vi "nanocal -- nuclear schottky fit -- 2x2 -- V9.vi"() -> ()   [LabVIEW 2021] (continued)
              n225 = for {
                tunnel: w525 -> [w532] mode=indexing
                tunnel: w524 -> [w533]
                tunnel: w523 -> [w531]
                tunnel: [w529] -> w522 mode=indexing
                n226 = Look In Map(map=w533, key=w532) -> (value=w530:string)  [unwired: 1 in, 1 out]
                n227 = Concatenate Strings(w531, w530) -> (w529:string)
              }
            }
            n228 = call "string parse mathematica list assosiated array -- V2.vi"("action"=3-lorentzian-heat-response_action."create emty string" ("derivative"), "array of IDs"=w519) -> ("string out"=w520:string)  [unwired: 8 in, 1 out]
            n229 = local write "string OUT"(w520) -> ()
          }
          frame "action: update enums" {
            w537 = map{string, string} {}  # Size: 0
            w543 = map{i32, string} {}  # Size: 0
            # "gives a key"
            n230 = local read "selector"() -> (w535:T10)
            n231 = local read "all short filenames"() -> (w538:map{string, string})
            n232 = in-place {
              w560 = map{i32, dbl} {}  # Size: 0
              w566 = map{i32, dbl} {}  # Size: 0
              w567 = map{i32, dbl} {}  # Size: 0
              w569 = map{i32, dbl} {}  # Size: 0
              w568 = map{i32, dbl} {}  # Size: 0
              n233 = in-place-cluster #4(w535) -> ("lookup.all set of"=w554:set{dbl}, "lookup.all sides"=w553:set{dbl}, "lookup.all T's"=w552:set{dbl}, "lookup.all θ's"=w551:set{dbl}, "lookup.all B's"=w550:set{dbl})  [unwired: 5 out]
              n234 = for {
                shift-right: [w573] -> w559
                shift-left: w560 -> [w574]
                tunnel: [w571] -> w561 mode=indexing
                tunnel: w554 -> [w570] mode=indexing
                i -> [w572]
                n235 = Number To Decimal String(number=w570) -> (decimal integer string=w571:string)  [unwired: 1 in]
                n236 = Insert Into Map(map in=w574, key=w572, value=w570) -> (map out=w573:map{i32, dbl})  [unwired: 2 out]
              }
              n237 = for {
                shift-right: [w584] -> w556
                shift-left: w567 -> [w585]
                tunnel: [w582] -> w563 mode=indexing
                tunnel: w552 -> [w581] mode=indexing
                i -> [w583]
                n238 = Number To Fractional String(number=w581, precision (6)=i16 3) -> (F-format string=w582:string)  [unwired: 2 in]
                n239 = Insert Into Map(map in=w585, key=w583, value=w581) -> (map out=w584:map{i32, dbl})  [unwired: 2 out]
              }
              n240 = property on="set (1T|2B)" class="Ring (strict)"("Strings []"=w561) -> ()  [unwired: 2 in, 2 out]
              n241 = property on="T (K)" class="Ring (strict)"("Strings []"=w563) -> ()  [unwired: 2 in, 2 out]
              n242 = for {
                shift-right: [w578] -> w558
                shift-left: w566 -> [w579]
                tunnel: [w576] -> w562 mode=indexing
                tunnel: w553 -> [w575] mode=indexing
                i -> [w577]
                n243 = Number To Decimal String(number=w575) -> (decimal integer string=w576:string)  [unwired: 1 in]
                n244 = Insert Into Map(map in=w579, key=w577, value=w575) -> (map out=w578:map{i32, dbl})  [unwired: 2 out]
              }
              n245 = for {
                shift-right: [w596] -> w555
                shift-left: w568 -> [w597]
                tunnel: [w594] -> w564 mode=indexing
                tunnel: w551 -> [w593] mode=indexing
                i -> [w595]
                n246 = Number To Fractional String(number=w593, precision (6)=i16 3) -> (F-format string=w594:string)  [unwired: 2 in]
                n247 = Insert Into Map(map in=w597, key=w595, value=w593) -> (map out=w596:map{i32, dbl})  [unwired: 2 out]
              }
              n248 = property on="side (8S|4R)" class="Ring (strict)"("Strings []"=w562) -> ()  [unwired: 2 in, 2 out]
              n249 = property on="θ (deg)" class="Ring (strict)"("Strings []"=w564) -> ()  [unwired: 2 in, 2 out]
              n250 = for {
                shift-right: [w590] -> w557
                shift-left: w569 -> [w591]
                tunnel: [w588] -> w565 mode=indexing
                tunnel: w550 -> [w587] mode=indexing
                i -> [w589]
                n251 = Number To Fractional String(number=w587, precision (6)=i16 3) -> (F-format string=w588:string)  [unwired: 2 in]
                n252 = Insert Into Map(map in=w591, key=w589, value=w587) -> (map out=w590:map{i32, dbl})  [unwired: 2 out]
              }
              n253 = property on="B (T)" class="Ring (strict)"("Strings []"=w565) -> ()  [unwired: 2 in, 2 out]
              n254 = in-place-cluster #4("lookup.all set of"=w554, "lookup.all sides"=w553, "lookup.all T's"=w552, "lookup.all θ's"=w551, "lookup.all B's"=w550, "lookup.set of lookup"=w559, "lookup.side lookup"=w558, "lookup.T lookup"=w556, "lookup.B lookup"=w557, "lookup.θ lookup"=w555) -> (w534:T10)
            }
            n255 = for {
              tunnel: w538 -> [w602] mode=indexing
              shift-right: [w600] -> w536
              shift-left: w537 -> [w601]
              n256 = Unbundle(w602) -> ("event data"=w598:string, "file pattern"=w599:string)
              n257 = Insert Into Map(map in=w601, key=w599, value=w598) -> (map out=w600:map{string, string})  [unwired: 2 out]
            }
            n258 = local read "temps&degs"() -> (w542:map{string, map{T2, dbl}})
            n259 = local read "X selector"() -> (w541:T2)
            n260 = for {
              tunnel: [w611] -> w546 mode=indexing
              tunnel: [w615] -> w544 mode=indexing
              tunnel: [w612] -> w548 mode=indexing
              tunnel: w541 -> [w616]
              tunnel: w536 -> [w614] mode=indexing
              tunnel: w542 -> [w613]
              n261 = Unbundle(w614) -> (w611:string, w612:string)
              n262 = Look In Map(map=w613, key=w612) -> (value=w617:map{T2, dbl})  [unwired: 1 in, 1 out]
              n263 = Look In Map(map=w617, key=w616) -> (value=w615:dbl)  [unwired: 1 in, 1 out]
            }
            n264 = call "array - sorted inexes.vi"("x"=w544) -> ("index array"=w545:i32[])  [unwired: 9 in, 1 out]
            n265 = for {
              tunnel: w545 -> [w607] mode=indexing
              tunnel: w546 -> [w610]
              tunnel: [w609] -> w547 mode=indexing
              tunnel: w548 -> [w608]
              shift-right: [w603] -> w549
              shift-left: w543 -> [w606]
              i -> [w605]
              n266 = Index Array(array=w610, index=w607) -> (element=w609:string)
              n267 = Index Array(array=w608, index=w607) -> (element=w604:string)
              n268 = Insert Into Map(map in=w606, key=w605, value=w604) -> (map out=w603:map{i32, string})  [unwired: 2 out]
            }
            "filesnames lookup" <- w549
            n269 = property on="filenames" class="Ring (strict)"("Strings []"=w547) -> ()  [unwired: 2 in, 2 out]
            n270 = Generate User Event(user event=w539, event data cluster="action: update state of selectors" ("event data")) -> ()  [unwired: 2 in, 2 out]
            n271 = local write "selector"(w534) -> ()
          }
          frame "action: update constrained file selector" {
            w624 = map{i32, string} {}  # Size: 0
            n272 = local read "state of all selectors"() -> (w620:map{T2, map{bool, dbl}})
            n273 = local read "all short filenames"() -> (w621:map{string, string})
            n274 = local read "temps&degs"() -> (w622:map{string, map{T2, dbl}})
            n275 = for {
              tunnel: w621 -> [w634] mode=indexing
              tunnel: [w634] -> w623 mode=indexing if=w630
              shift-right: [w633] -> w619
              shift-left: w622 -> [w633]
              tunnel: w620 -> [w631]
              n276 = for {
                tunnel: [w646] -> w632 mode=indexing
                shift-right: [w641] -> _
                shift-left: w634 -> [w641]
                shift-right: [w640] -> _
                shift-left: w633 -> [w640]
                tunnel: w631 -> [w639] mode=indexing
                n277 = Unbundle(w641) -> ("event data"=w645:string)  [unwired: 1 out]
                n278 = Unbundle(w639) -> ("Plost: sweep window"=w638:T2, "map"=w637:map{bool, dbl})
                n279 = for {
                  tunnel: w637 -> [w649] mode=indexing
                  tunnel: [w648] -> w635
                  tunnel: [w647] -> w636
                  n280 = Unbundle(w649) -> ("ignore side !"=w648:bool, "number OUT"=w647:dbl)
                }
                n281 = Look In Map(map=w640, key=w645) -> (value=w644:map{T2, dbl})  [unwired: 1 in, 1 out]
                n282 = Look In Map(map=w644, key=w638) -> (value=w643:dbl)  [unwired: 1 in, 1 out]
                n283 = Equal?(x=w643, y=w636) -> (x = y?=w642:bool)
                n284 = Or(x=w635, y=w642) -> (x .or. y?=w646:bool)
              }
              n285 = And Array Elements(Boolean array=w632) -> (logical AND=w630:bool)
            }
            n286 = for {
              tunnel: [w664] -> w627 mode=indexing
              tunnel: [w662] -> w625 mode=indexing
              tunnel: [w659] -> w629 mode=indexing
              tunnel: w623 -> [w661] mode=indexing
              tunnel: w619 -> [w660]
              n287 = Unbundle(w661) -> ("event data"=w659:string, "file pattern"=w664:string)
              n288 = local read "X selector"() -> (w658:T2)
              n289 = Look In Map(map=w660, key=w659) -> (value=w663:map{T2, dbl})  [unwired: 1 in, 1 out]
              n290 = Look In Map(map=w663, key=w658) -> (value=w662:dbl)  [unwired: 1 in, 1 out]
            }
            n291 = call "array - sorted inexes.vi"("x"=w625) -> ("index array"=w626:i32[])  [unwired: 9 in, 1 out]
            n292 = for {
              tunnel: w626 -> [w654] mode=indexing
              tunnel: w627 -> [w657]
              tunnel: [w656] -> w628 mode=indexing
              tunnel: w629 -> [w655]
              shift-right: [w650] -> w618
              shift-left: w624 -> [w653]
              i -> [w652]
              n293 = Index Array(array=w657, index=w654) -> (element=w656:string)
              n294 = Index Array(array=w655, index=w654) -> (element=w651:string)
              n295 = Insert Into Map(map in=w653, key=w652, value=w651) -> (map out=w650:map{i32, string})  [unwired: 2 out]
            }
            "constrained filename lookup" <- w618
            n296 = property on="selection :|\\" class="Ring (strict)"("Strings []"=w628) -> ()  [unwired: 2 in, 2 out]
          }
          frame "action: constrained filenames select" {
            (unwired) 1
            n297 = local read "constrained filename lookup"() -> (w667:map{i32, string})
            n298 = local read "selection :|\\"() -> (w668:u16)
            n299 = local read "all full filenames"() -> (w669:map{string, path})
            n300 = Look In Map(map=w667, key=w668) -> (value=w670:string)  [unwired: 1 in, 1 out]
            n301 = Look In Map(map=w669, key=w670) -> (value=w671:path)  [unwired: 1 in, 1 out]
            n302 = local write "Read from file"(w671) -> ()
            n303 = Generate User Event(user event=w666, event data cluster="action: read from file" ("event data")) -> ()  [unwired: 2 in, 2 out]
          }
          frame "action: write mathematica string" {
            n304 = local read "mathematica thing"() -> (w676:map{string, map{T2, dbl}})
            n305 = local read "folder"() -> (w675:path)
            n306 = Build Path(base path=w675, name or relative path="temporarystring.txt") -> (appended path=w674:path)
            n307 = call "string parse mathematica list assosiated array -- V2.vi"("action"=3-lorentzian-heat-response_action."create string" ("derivative"), "Map IN"=w676) -> ("string out"=w672:string)  [unwired: 8 in, 1 out]
            "string OUT" <- w672
            n308 = Write to Text File(file (use dialog)=w674, text=w672) -> ()  [unwired: 2 in, 3 out]
          }
          frame "action: replot colors" {
            # "all -- including kappa0"
            n309 = local read "state of all selectors string"() -> (w687:string)
            n310 = local read "new selector names"() -> (w692:map{T2, map{T19, string}})
            n311 = local read "X selector"() -> (w688:T2)
            n312 = Build Array (concatenate)(w680, w678) -> (w679:T2[])
            n313 = local read "state of all selectors"() -> (w699:map{T2, map{bool, dbl}})
            n314 = Look In Map(map=w692, key=w688) -> (value=w691:map{T19, string})  [unwired: 1 in, 1 out]
            n315 = local read "mathematica thing"() -> (w700:map{string, map{T2, dbl}})
            n316 = Look In Map(map=w691, key=nameformattingitem."nameL") -> (value=w689:string)  [unwired: 1 in, 1 out]
            n317 = Concatenate Strings(w687, w689) -> (w698:string)
            n318 = for {
              tunnel: w700 -> [w721]
              tunnel: w688 -> [w716]
              tunnel: w679 -> [w704] mode=indexing
              tunnel: w699 -> [w717]
              tunnel: w692 -> [w708]
              shift-right: [w712] -> w686
              shift-left: w698 -> [w715]
              tunnel: w687 -> [w713]
              tunnel: [w709] -> w685 mode=indexing
              n319 = for {
                tunnel: w721 -> [w735] mode=indexing
                tunnel: w704 -> [w734]
                tunnel: [w733] -> w720 mode=indexing if=w727
                tunnel: [w732] -> w719 mode=indexing if=w727
                tunnel: w716 -> [w731]
                tunnel: w717 -> [w730]
                n320 = Unbundle(w735) -> ("Map"=w729:map{T2, dbl})  [unwired: 1 out]
                n321 = for {
                  tunnel: w730 -> [w744] mode=indexing
                  tunnel: w729 -> [w743]
                  tunnel: [w741] -> w728 mode=indexing
                  n322 = Unbundle(w744) -> ("Plost: sweep window"=w742:T2, "map"=w740:map{bool, dbl})
                  n323 = for {
                    tunnel: w740 -> [w747] mode=indexing
                    tunnel: [w746] -> w737
                    tunnel: [w745] -> w738
                    n324 = Unbundle(w747) -> ("ignore side !"=w746:bool, "number OUT"=w745:dbl)
                  }
                  n325 = Look In Map(map=w743, key=w742) -> (value=w739:dbl)  [unwired: 1 in, 1 out]
                  n326 = Equal?(x=w739, y=w738) -> (x = y?=w736:bool)
                  n327 = Or(x=w737, y=w736) -> (x .or. y?=w741:bool)
                }
                n328 = Look In Map(map=w729, key=w731) -> (value=w733:dbl)  [unwired: 1 in, 1 out]
                n329 = Look In Map(map=w729, key=w734) -> (value=w732:dbl)  [unwired: 1 in, 1 out]
                n330 = And Array Elements(Boolean array=w728) -> (logical AND=w727:bool)
              }
              n331 = Look In Map(map=w708, key=w704) -> (value=w706:map{T19, string})  [unwired: 1 in, 1 out]
              n332 = Look In Map(map=w706, key=nameformattingitem."nameL") -> (value=w705:string)  [unwired: 1 in, 1 out]
              n333 = call <vilib>:"Space Constant.vi"() -> ("String"=w714:string)
              n334 = Concatenate Strings(w715, w714, w713, w705) -> (w712:string)
              n335 = call "array - sorted inexes.vi"("x"=w720) -> ("index array"=w718:i32[])  [unwired: 9 in, 1 out]
              n336 = for {
                tunnel: w720 -> [w726]
                tunnel: w719 -> [w725]
                tunnel: w718 -> [w722] mode=indexing
                tunnel: [w724] -> w711 mode=indexing
                tunnel: [w723] -> w710 mode=indexing
                n337 = Index Array(array=w726, index=w722) -> (element=w724:dbl)
                n338 = Index Array(array=w725, index=w722) -> (element=w723:dbl)
              }
              n339 = Bundle(w711, w710) -> (w709:cluster{dbl[], dbl[]})  [unwired: 1 in]
            }
            n340 = local read "folder"() -> (w697:path)
            n341 = Concatenate Strings("plotstring", w687, ".dat") -> (w693:string)
            n342 = Build Path(base path=w697, name or relative path=w693) -> (appended path=w696:path)
            n343 = call "nanocal -- plotstring file manage.vi"("Enum"=nanocal_--_plotstring_file_action."generate plotstring thing", "all data"=w685, "header line"=w686) -> ("plotstring thing"=w683:string)  [unwired: 8 in]
            n344 = flat-sequence {
              tunnel: w685 -> [w701]
              tunnel: w682 -> [w703]
              tunnel: "interface: replot colors plot" ("event data") -> [w702]
              frame #0 {
                "color data" <- w701
              }
              frame #1 {
                n345 = Generate User Event(user event=w703, event data cluster=w702) -> ()  [unwired: 2 in, 2 out]
              }
            }
            n346 = Write to Text File(file (use dialog)=w696, text=w683) -> ()  [unwired: 2 in, 3 out]
          }
          frame "action: update state of selectors" {
            w768 = T2[] [enum."T (K)", enum."B (T)", enum."θ (deg)", enum."side (S|R)"] items=["ζ", "τ1", "τS", "τN", "τC", "κ0", "m1", "m2", "m3", "T (K)", "B (T)", "θ (deg)", "side (S|R)", "set of (B|T)", "Re(offset)", "Im(offset)", "στ1", "στ1-", "στ1+", "στS", "στS-", "στS+", "στN", "στN-", "στN+", "τ11", "τ12", "τ21", "τ22", "τN1", "τN2"]  # selector fields
            n347 = local read "selector"() -> (w764:T10)
            n348 = Unbundle By Name(w764) -> ("side (8S|4R)"=w763:i32, "ignore side !"=w762:bool, "lookup.side lookup"=w761:map{i32, dbl}, "T (K)"=w758:u16, "ignore T !"=w760:bool, "lookup.T lookup"=w759:map{i32, dbl}, "B (T)"=w755:u16, "ignore B !"=w757:bool, "lookup.B lookup"=w756:map{i32, dbl}, "θ (deg)"=w753:u16, "ignore θ !"=w752:bool, "lookup.θ lookup"=w754:map{i32, dbl}, "set (1T|2B)"=w749:i32, "ignore set of !"=w750:bool, "lookup.set of lookup"=w751:map{i32, dbl})
            n349 = Look In Map(map=w761, key=w763) -> (value=w767:dbl)  [unwired: 1 in, 1 out]
            n350 = local read "new selector names"() -> (w771:map{T2, map{T19, string}})
            n351 = node(w762, w767) -> (w788:map{bool, dbl})
            n352 = Look In Map(map=w759, key=w758) -> (value=w787:dbl)  [unwired: 1 in, 1 out]
            n353 = Look In Map(map=w756, key=w755) -> (value=w783:dbl)  [unwired: 1 in, 1 out]
            n354 = node(w760, w787) -> (w785:map{bool, dbl})
            n355 = node(w757, w783) -> (w782:map{bool, dbl})
            n356 = Look In Map(map=w754, key=w753) -> (value=w781:dbl)  [unwired: 1 in, 1 out]
            n357 = node(w752, w781) -> (w779:map{bool, dbl})
            n358 = Look In Map(map=w751, key=w749) -> (value=w778:dbl)  [unwired: 1 in, 1 out]
            n359 = node(w750, w778) -> (w776:map{bool, dbl})
            n360 = local read "side map from NUM"() -> (w765:map{i32, T8})
            n361 = node(3-lorentzian-parameters."side (S|R)" ("Plost: sweep window"), w788, 3-lorentzian-parameters."T (K)" ("Plost: sweep window"), w785, 3-lorentzian-parameters."B (T)" ("Plost: sweep window"), w782, 3-lorentzian-parameters."θ (deg)" ("Plost: sweep window"), w779, 3-lorentzian-parameters."set of (B|T)" ("Plost: sweep window"), w776) -> (w748:map{T2, map{bool, dbl}})
            "state of all selectors" <- w748
            n362 = for {
              tunnel: w771 -> [w793]
              shift-right: [w796] -> w769
              shift-left: "_" ("event data") -> [w795]
              tunnel: w768 -> [w792] mode=indexing
              tunnel: w748 -> [w790]
              n363 = Look In Map(map=w790, key=w792) -> (value=w798:map{bool, dbl})  [unwired: 1 in, 1 out]
              n364 = Look In Map(map=w793, key=w792) -> (value=w791:map{T19, string})  [unwired: 1 in, 1 out]
              n365 = for {
                tunnel: w798 -> [w813] mode=indexing
                tunnel: [w812] -> w797
                tunnel: [w811] -> w794
                n366 = Unbundle(w813) -> ("ignore side !"=w812:bool, "number OUT"=w811:dbl)
              }
              n367 = case shown="False" w797 {
                tunnel: [w809 w810] -> w796
                tunnel: w795 -> [w808 w810]
                tunnel: w794 -> [w805 _]
                tunnel: w791 -> [w801 _]
                frame False {
                  n368 = Look In Map(map=w801, key=nameformattingitem."units") -> (value=w802:string)  [unwired: 1 in, 1 out]
                  n369 = Look In Map(map=w801, key=nameformattingitem."prec") -> (value=w799:string)  [unwired: 1 in, 1 out]
                  n370 = Format Value(format string=w799, value (0)=w805) -> (output string=w804:string)  [unwired: 1 in]
                  n371 = Concatenate Strings(w808, "_" ("event data"), w804, w802, "_" ("event data")) -> (w809:string)
                }
                frame True {
                }
              }
            }
            "state of all selectors string" <- w769
            n372 = Look In Map(map=w765, key=w767) -> (value=w766:T8)  [unwired: 1 in, 1 out]
            n373 = local write "side"(w766) -> ()
            n374 = Generate User Event(user event=w772, event data cluster="action: replot colors" ("event data")) -> (user event out=w773:refnum<user-event>)  [unwired: 2 in, 1 out]
            n375 = Generate User Event(user event=w773, event data cluster="action: update constrained file selector" ("event data")) -> ()  [unwired: 2 in, 2 out]
          }
          frame "action: copy from math" {
            w823 = map{T2, bool} {}  # Size: 0
            n376 = local read "defaults selector"() -> (w822:T9)
            n377 = local read "mathematica thing"() -> (w828:map{string, map{T2, dbl}})
            n378 = case shown="True" "overwrite offset" {
              tunnel: w820 -> [w831 w835]
              tunnel: [w831 w834] -> w819
              frame False {
              }
              frame True {
                n379 = Build Array (concatenate)(w835, 3-lorentzian-parameters."Re(offset)" ("Plost: sweep window"), 3-lorentzian-parameters."Im(offset)" ("Plost: sweep window")) -> (w834:T2[])
              }
            }
            n380 = for {
              shift-right: [w839] -> w821
              shift-left: w823 -> [w840]
              tunnel: w822 -> [w838] mode=indexing
              n381 = Unbundle(w838) -> ("Plost: sweep window"=w837:T2, "used default"=w836:bool)
              n382 = Insert Into Map(map in=w840, key=w837, value=w836) -> (map out=w839:map{T2, bool})  [unwired: 2 out]
            }
            n383 = local read "key"() -> (w827:string)
            n384 = local read "parameter map"() -> (w816:map{T2, dbl})
            n385 = Look In Map(map=w828, key=w827) -> (key not found?=w825:bool, value=w826:map{T2, dbl})  [unwired: 1 in]
            n386 = case shown="False" w825 {
              tunnel: w826 -> [w855 _]
              tunnel: w821 -> [w853 _]
              tunnel: w819 -> [w854 _]
              tunnel: "overwrite offset" -> [w847 w892]
              tunnel: [w846 w892] -> w817
              tunnel: w816 -> [w845 _]
              tunnel: w814 -> [w843 _]
              frame False {
                # "the order of numbers \nMUST corrspond to order\nin the \"parameter\" array"
                n387 = for {
                  tunnel: [w867] -> w852 mode=indexing
                  tunnel: w855 -> [w875]
                  tunnel: w854 -> [w868] mode=indexing
                  tunnel: w853 -> [w874]
                  shift-right: [w869] -> w844
                  shift-left: w845 -> [w870]
                  n388 = Look In Map(map=w874, key=w868, default value=FALSE) -> (value=w873:bool)  [unwired: 1 out]
                  n389 = Look In Map(map=w875, key=w868) -> (value=w872:dbl)  [unwired: 1 in, 1 out]
                  n390 = case shown="True" w873 {
                    tunnel: w872 -> [w878 _]
                    tunnel: w868 -> [_ w879]
                    tunnel: [w878 w880] -> w867
                    frame False {
                    }
                    frame True {
                      n391 = local read "T (K)"() -> (w891:dbl)
                      n392 = local read "B (T)"() -> (w887:dbl)
                      n393 = Divide(x=w887, y=12.0) -> (x/y=w885:dbl)
                      n394 = Equal?(x=3-lorentzian-parameters."τN", y=w879) -> (x = y?=w888:bool)
                      n395 = Square(x=w885) -> (x^2=w884:dbl)
                      n396 = call "nanocal -- defaut parameter manager -- V1.vi"("action"=nanocal_--_defaut_parameter_manager_action--_V1."get logarithmic interp", "T"=w891, "what"=w879) -> ("number"=w882:dbl)  [unwired: 8 in]
                      n397 = Select(t=w884, s=w888, f=1.0) -> (s? t:f=w881:dbl)
                      n398 = Multiply(x=w882, y=w881) -> (x*y=w880:dbl)
                    }
                  }
                  n399 = in-place {
                    in-place-border: w867 -> [w877]
                    in-place-border: LVMapReplaceAction."Modify Entry only if found" ("action") -> [w876]
                    n400 = in-place-map #5(w870, w868) -> ()  [unwired: 1 in, 2 out]
                    n401 = in-place-map #5(w877, w876) -> (w869:map{T2, dbl})  [unwired: 2 out]
                  }
                }
                n402 = Index Array(array=w852, index #1=6 ("index"), index #2=7 ("index")) -> (element #1=w849:dbl, element #2=w848:dbl)
                n403 = flat-sequence {
                  tunnel: w844 -> [w856]
                  tunnel: w843 -> [w860]
                  tunnel: "interface: update list from parameter map" ("event data") -> [w859]
                  tunnel: "interface: update curvature plot" ("event data") -> [w857]
                  frame #0 {
                    n404 = local write "parameter map"(w856) -> ()
                  }
                  frame #1 {
                    n405 = Generate User Event(user event=w860, event data cluster=w859) -> (user event out=w858:refnum<user-event>)  [unwired: 2 in, 1 out]
                    n406 = Generate User Event(user event=w858, event data cluster=w857) -> ()  [unwired: 2 in, 2 out]
                  }
                }
                n407 = case shown="True" w847 {
                  selector: w847 -> [w861 w862]
                  tunnel: w849 -> [_ w864]
                  tunnel: w848 -> [_ w863]
                  tunnel: [w861 w862] -> w846
                  frame False {
                  }
                  frame True {
                    n408 = Bundle("number"=w864, "number"=w863) -> (w865:cluster{"number":dbl, "number":dbl})  [unwired: 1 in]
                    n409 = local write "offset Re\noffset Im"(w865) -> ()
                  }
                }
              }
              frame True {
              }
            }
            n410 = case shown="True" w817 {
              tunnel: ["action: new sweep" ("event data") "action: read from file" ("event data")] -> w815
              frame False {
              }
              frame True {
              }
            }
            n411 = Generate User Event(user event=w824, event data cluster=w815) -> ()  [unwired: 2 in, 2 out]
          }
          frame "action: copy to math" {
            n412 = local read "error goodness weighting"() -> (w904:T5)
            n413 = local read "offset Re\noffset Im"() -> (w915:cluster{"Numeric":dbl, "Numeric":dbl})
            n414 = local read "newton parameters"() -> (w906:T3)
            n415 = local read "sampling size(%)"() -> (w908:dbl)
            n416 = local read "curvature triplets"() -> (w910:T11[])
            n417 = local read "parameter map"() -> (w911:map{T2, dbl})
            n418 = local read "error-mode"() -> (w894:T15)
            n419 = call "nanocal -- publish -- freq scan V2.vi"("publisher action"=publisher_action."get") -> ("data"=w909:T34)  [unwired: 7 in, 3 out]
            n420 = local read "parameter map"() -> (w912:map{T2, dbl})
            n421 = local read "θ (deg)"() -> (w919:dbl)
            n422 = Build Array (concatenate)(w893, w896) -> (w895:T2[])
            n423 = local read "T (K)"() -> (w921:dbl)
            n424 = local read "B (T)"() -> (w920:dbl)
            n425 = Unbundle(w915) -> ("Numeric"=w914:dbl, "Numeric"=w913:dbl)
            n426 = Bundle By Name(cluster=w906, "weighting"=w904) -> (w905:T3)
            n427 = Build Array(w921, w920, w919, w914, w913) -> (w903:dbl[])
            n428 = call "nanocal -- generate 3D curvature ellipsoid --  V4.vi"("sampling vicinity size (%)"=w908, "error mode"=w894, "newton parameters"=w905, "data"=w909, "Curvature triplet array IN"=w910, "parameter map"=w911) -> ("Curvature triplet array OUT"=w900:T11[])  [unwired: 5 in]
            n429 = local write "curvature triplets"(w900) -> ()
            n430 = Index Array(array=w900, index=0) -> (element=w898:T11)
            n431 = Unbundle By Name(w898) -> ("pars & errors"=w897:map{T2, dbl})
            n432 = for {
              tunnel: w896 -> [w929] mode=indexing
              shift-right: [w930] -> _
              shift-left: w897 -> [w930]
              tunnel: [w928] -> w902 mode=indexing
              n433 = Look In Map(map=w930, key=w929, default value=0.0) -> (value=w928:dbl)  [unwired: 1 out]
            }
            n434 = Build Array (concatenate)(w903, w902) -> (w901:dbl[])
            n435 = for {
              tunnel: w901 -> [w931] mode=indexing
              tunnel: w895 -> [w932] mode=indexing
              shift-right: [w933] -> w918
              shift-left: w912 -> [w934]
              n436 = Insert Into Map(map in=w934, key=w932, value=w931) -> (map out=w933:map{T2, dbl})  [unwired: 2 out]
            }
            n437 = local read "mathematica thing"() -> (w924:map{string, map{T2, dbl}})
            n438 = local read "key"() -> (w923:string)
            n439 = call "3-lorentzian-heat-response -- V4.vi"("action"=3-lorentzian-heat-response_action."calc m1m2m3", "Map IN"=w918) -> ("Map OUT"=w917:map{T2, dbl})  [unwired: 7 in, 2 out]
            n440 = in-place {
              in-place-border: w917 -> [w935]
              n441 = in-place-map #6(w924, w923) -> (w938:map{T2, dbl})  [unwired: 1 in, 1 out]
              n442 = for {
                tunnel: w935 -> [w940] mode=indexing
                shift-right: [w943] -> w937
                shift-left: w938 -> [w944]
                shift-right: [w942] -> _
                shift-left: w935 -> [w942]
                n443 = Unbundle(w940) -> ("X selector"=w939:T2)  [unwired: 1 out]
                n444 = Look In Map(map=w942, key=w939) -> (value=w941:dbl)  [unwired: 1 in, 1 out]
                n445 = Insert Into Map(map in=w944, key=w939, value=w941) -> (map out=w943:map{T2, dbl})  [unwired: 2 out]
              }
              n446 = in-place-map #6(w937, LVMapReplaceAction."Modify Entry only if found" ("action")) -> (w922:map{string, map{T2, dbl}})  [unwired: 2 out]
            }
            n447 = local write "mathematica thing"(w922) -> ()
            n448 = Generate User Event(user event=w925, event data cluster="action: replot colors" ("event data")) -> ()  [unwired: 2 in, 2 out]
          }
          frame "action: exit" {
          }
          frame "action: read from file" {
            n449 = local read "Read from file"() -> (w946:path)
            n450 = local read "cursor x selector"() -> (w969:map{T2, dbl})
            n451 = call "file - read-write - list of lines-V2.vi"("read/write control"=file_--_read-write_control."read", "file path"=w946) -> ("header OUT"=w956:string, "list of lines OUT"=w958:string[], "filename out"=w986:string)  [unwired: 7 in]
            n452 = Unbundle("offset Re\noffset Im") -> ("Numeric"=w972:dbl, "Numeric"=w971:dbl)
            n453 = call "filename-manage.vi"("filename-action"=filename-action."get name", "file name IN"=w986) -> ("string OUT"=w955:string)  [unwired: 7 in, 2 out]
            n454 = Re/Im To Complex(1:w971, 2:w972) -> (0:w959:cdb)
            n455 = call "filename-manage.vi"("filename-action"=filename-action."get T", "file name IN"=w955) -> ("number OUT"=w968:dbl, "filename OUT"=w983:string)  [unwired: 7 in, 1 out]
            "T (K)" <- w968
            n456 = case shown="\"raw nanocal\"" "data file formatting" {
              tunnel: [w992 w1006 w1050 w1077] -> w980
              tunnel: [w991 w1005 w1049 w1076] -> w974
              tunnel: w959 -> [w990 w1014 w1045 w1066]
              tunnel: w958 -> [w993 w1018 w1044 w1065]
              tunnel: w956 -> [_ w1019 _ _]
              tunnel: w955 -> [_ w1012 _ _]
              tunnel: w946 -> [_ w1013 _ _]
              tunnel: "side" -> [_ w1011 _ _]
              tunnel: "toggle generate labview files" -> [_ w1009 _ _]
              frame "as is", Default {
                n457 = for {
                  tunnel: w993 -> [w1004] mode=indexing
                  tunnel: [w999] -> w994 mode=indexing if=w995
                  tunnel: [w998] -> w992 mode=indexing if=w995
                  w1000 = 0.0
                  n458 = Scan From String(format string="%f%f%f", input string=w1004, initial scan location=u32 0, default 1=w1000, default 2=w1000, default 3=w1000) -> (offset past scan=w996:u32, output 1=w998:dbl, output 2=w1002:dbl, output 3=w1001:dbl)  [unwired: 1 in, 2 out]
                  n459 = Greater Than 0?(x=w996) -> (x > 0?=w995:bool)
                  n460 = Re/Im To Complex(1:w1001, 2:w1002) -> (0:w999:cdb)
                }
                n461 = Subtract(x=w994, y=w990) -> (x-y=w991:cdb[])
              }
              frame "raw nanocal" {
                w1008 = T32[] [enum."add -ω", enum."sort ω", enum."select |ω|<max"] items=["as is", "add -ω", "sort ω", "2 x ω", "R-phase(deg) to Re-Im", "select ω>0", "labview file str", "select |ω|<max"]
                n462 = case shown="\"ref\"" w1011 {
                  tunnel: [nanocal_raw_file_manage_action_V1."read S side" ("action") nanocal_raw_file_manage_action_V1."read R side" ("action")] -> w1010
                  frame "sam", Default {
                  }
                  frame "ref" {
                  }
                }
                n463 = call "nanocal_raw_file_manage_V1.vi"("action"=w1010, "list of lines IN"=w1018, "header IN"=w1019) -> ("z (K/W)  OUT"=w1015:cdb[], "f (Hz) OUT"=w1016:dbl[])  [unwired: 6 in, 1 out]
                n464 = Subtract(x=w1015, y=w1014) -> (x-y=w1017:cdb[])
                n465 = for {
                  shift-right: [w1023] -> w1006
                  shift-left: w1016 -> [w1024]
                  shift-right: [w1022] -> w1005
                  shift-left: w1017 -> [w1025]
                  tunnel: w1008 -> [w1021] mode=indexing
                  tunnel: "|ω| < limit (Hz)" -> [w1020]
                  n466 = call "array -- freq-voltage transformations.vi"("number"=w1020, "freq voltage action"=w1021, "z In"=w1025, "ω IN"=w1024) -> ("z out"=w1022:cdb[], "ω out"=w1023:dbl[])  [unwired: 4 in, 2 out]
                }
                n467 = case shown="True" w1009 {
                  tunnel: w1013 -> [_ w1037]
                  tunnel: w1012 -> [_ w1041]
                  tunnel: w1006 -> [_ w1033]
                  tunnel: w1005 -> [_ w1032]
                  frame False {
                  }
                  frame True {
                    n468 = call "filename-manage.vi"("filename-action"=filename-action."get basename", "file name IN"=w1041) -> ("string OUT"=w1039:string)  [unwired: 7 in, 2 out]
                    n469 = Strip Path(path=w1037) -> (stripped path=w1036:path)  [unwired: 1 out]
                    n470 = Concatenate Strings(w1039, "_labview_.dat") -> (w1028:string)
                    n471 = call "array -- freq-voltage transformations.vi"("freq voltage action"=array_--_freq-voltage_transformations_action."labview file str", "z In"=w1032, "ω IN"=w1033) -> ("lines out"=w1030:string[], "header OUT"=w1031:string)  [unwired: 5 in, 2 out]
                    n472 = Build Path(base path=w1036, name or relative path=w1028) -> (appended path=w1035:path)
                    n473 = call "file - read-write - list of lines-V2.vi"("read/write control"=file_--_read-write_control."write all", "header IN"=w1031, "list of lines IN"=w1030, "file path"=w1035) -> ()  [unwired: 5 in, 3 out]
                  }
                }
              }
              frame "add - ω" {
                n474 = for {
                  tunnel: w1044 -> [w1062] mode=indexing
                  tunnel: [w1057] -> w1046 mode=indexing if=w1053
                  tunnel: [w1056] -> w1042 mode=indexing if=w1053
                  w1058 = 0.0
                  n475 = Scan From String(format string="%f%f%f", input string=w1062, initial scan location=u32 0, default 1=w1058, default 2=w1058, default 3=w1058) -> (offset past scan=w1054:u32, output 1=w1056:dbl, output 2=w1060:dbl, output 3=w1059:dbl)  [unwired: 1 in, 2 out]
                  n476 = Greater Than 0?(x=w1054) -> (x > 0?=w1053:bool)
                  n477 = Re/Im To Complex(1:w1059, 2:w1060) -> (0:w1057:cdb)
                }
                n478 = Subtract(x=w1046, y=w1045) -> (x-y=w1043:cdb[])
                n479 = call "array -- freq-voltage transformations.vi"("freq voltage action"=array_--_freq-voltage_transformations_action."add -ω", "z In"=w1043, "ω IN"=w1042) -> ("z out"=w1051:cdb[], "ω out"=w1052:dbl[])  [unwired: 5 in, 2 out]
                n480 = call "array -- freq-voltage transformations.vi"("freq voltage action"=array_--_freq-voltage_transformations_action."sort ω", "z In"=w1051, "ω IN"=w1052) -> ("z out"=w1049:cdb[], "ω out"=w1050:dbl[])  [unwired: 5 in, 2 out]
              }
              frame "full rydh" {
                n481 = for {
                  tunnel: w1065 -> [w1089] mode=indexing
                  tunnel: [w1084] -> w1067 mode=indexing if=w1080
                  tunnel: [w1083] -> w1063 mode=indexing if=w1080
                  w1085 = 0.0
                  n482 = Scan From String(format string="%f%f%f", input string=w1089, initial scan location=u32 0, default 1=w1085, default 2=w1085, default 3=w1085) -> (offset past scan=w1081:u32, output 1=w1083:dbl, output 2=w1087:dbl, output 3=w1086:dbl)  [unwired: 1 in, 2 out]
                  n483 = Greater Than 0?(x=w1081) -> (x > 0?=w1080:bool)
                  n484 = Re/Im To Complex(1:w1086, 2:w1087) -> (0:w1084:cdb)
                }
                n485 = Subtract(x=w1067, y=w1066) -> (x-y=w1064:cdb[])
                n486 = call "array -- freq-voltage transformations.vi"("freq voltage action"=array_--_freq-voltage_transformations_action."2 x ω", "z In"=w1064, "ω IN"=w1063) -> ("z out"=w1071:cdb[], "ω out"=w1073:dbl[])  [unwired: 5 in, 2 out]
                n487 = call "array -- freq-voltage transformations.vi"("freq voltage action"=array_--_freq-voltage_transformations_action."R-phase(deg) to Re-Im", "z In"=w1071, "ω IN"=w1073) -> ("z out"=w1070:cdb[], "ω out"=w1072:dbl[])  [unwired: 5 in, 2 out]
                n488 = call "array -- freq-voltage transformations.vi"("freq voltage action"=array_--_freq-voltage_transformations_action."add -ω", "z In"=w1070, "ω IN"=w1072) -> ("z out"=w1078:cdb[], "ω out"=w1079:dbl[])  [unwired: 5 in, 2 out]
                n489 = call "array -- freq-voltage transformations.vi"("freq voltage action"=array_--_freq-voltage_transformations_action."sort ω", "z In"=w1078, "ω IN"=w1079) -> ("z out"=w1076:cdb[], "ω out"=w1077:dbl[])  [unwired: 5 in, 2 out]
              }
            }
            n490 = Insert Into Map(map in=w969, key=3-lorentzian-parameters."T (K)" ("Plost: sweep window"), value=w968) -> (map out=w967:map{T2, dbl})  [unwired: 2 out]
            n491 = call "filename-manage.vi"("filename-action"=filename-action."get deg", "file name IN"=w983) -> ("number OUT"=w964:dbl, "filename OUT"=w950:string)  [unwired: 7 in, 1 out]
            "θ (deg)" <- w964
            n492 = Insert Into Map(map in=w967, key=3-lorentzian-parameters."θ (deg)" ("Plost: sweep window"), value=w964) -> (map out=w966:map{T2, dbl})  [unwired: 2 out]
            n493 = call "filename-manage.vi"("filename-action"=filename-action."get B", "file name IN"=w950) -> ("number OUT"=w963:dbl, "filename OUT"=w949:string)  [unwired: 7 in, 1 out]
            "B (T)" <- w963
            n494 = Insert Into Map(map in=w966, key=3-lorentzian-parameters."B (T)" ("Plost: sweep window"), value=w963) -> (map out=w965:map{T2, dbl})  [unwired: 2 out]
            n495 = local write "cursor x selector"(w965) -> ()
            n496 = local read "side map to STR"() -> (w948:map{T8, string})
            n497 = call "filename-manage.vi"("filename-action"=filename-action."getIDStock", "file name IN"=w949) -> ("string OUT"=w953:string)  [unwired: 7 in, 2 out]
            "file IDS" <- w953
            n498 = Look In Map(map=w948, key="side") -> (value=w954:string)  [unwired: 1 in, 1 out]
            n499 = Concatenate Strings(w953, w954) -> (→"key":string)
            n500 = call "filter - complex - four.vi"("omega (Hz) in"=w980, "z in"=w974, "span"="cspan") -> ("omega out"=w979:dbl[], "z out"=w978:cdb[], "dz/domega out"=w977:cdb[])  [unwired: 9 in, 5 out]
            n501 = call "nanocal -- publish -- freq scan V2.vi"("publisher action"=publisher_action."set", "dz/dω IN (V)"=w977, "z IN (V)"=w978, "ω IN (Hz)"=w979) -> ()  [unwired: 4 in, 4 out]
            n502 = Generate User Event(user event=w987, event data cluster="action: new sweep" ("event data")) -> ()  [unwired: 2 in, 2 out]
          }
          frame "action: save freq scan" {
            n503 = local read "Freq sweep name template"() -> (w1095:T7)
            n504 = call "MFLI -- publish -- freq scan.vi"("publisher action"=publisher_action."get") -> ("Voltage out (V)"=w1091:cdb[], "Freq out (Hz)"=w1092:dbl[])  [unwired: 9 in]
            n505 = call "filename-manage.vi"("filename pattern"=w1095, "filename-action"=filename-action."uniquenum", "folder IN"="Save folder", "file name IN"="freq sweep file name") -> ("filename OUT"=w1094:string)  [unwired: 5 in, 2 out]
            n506 = call "KM_appendline -- freq sweep.vi"("freq"=w1092, "Vout(V)"=w1091, "Save frequency scan"="Save folder", "read/write control"=KM_file_--_read-write_control."append one line", "name or relative path"=w1094) -> ()  [unwired: 15 in]
            n507 = local write "freq sweep file name"(w1094) -> ()
          }
          frame "void", Default {
          }
        }
      }
    }
  }
  n508 = while "interface actions" {
    tunnel: w11 -> [w1102]
    tunnel: w8 -> [w1101]
    tunnel: w7 -> [w1100]
    stop <- FALSE stop-if-true
    n509 = event shown="[0] <interface>: User Event" {
      selector: w1102 -> [_]
      dyn-events: _ -> [_]
      timeout: _ -> [_]
      tunnel: w1101 -> [w1104]
      tunnel: w1100 -> [w1103]
      event User Event {
        n510 = event-data() -> ("interface"=w1105:string)  [unwired: 1 in]
        n511 = case shown="\"interface: update curvature plot\"" w1105 {
          tunnel: [_ _ _ _ _ _ _ _ _ _ TRUE] -> _
          tunnel: w1104 -> [_ _ w1126 w1158 _ _ w1219 w1250 _ _ _]
          tunnel: w1103 -> [_ _ _ _ w1176 _ _ _ _ _ _]
          frame "void", Default {
          }
          frame "interface: reset colors" {
            w1112 = map{T2, u32} {}  # Size: 0
            n512 = local read "parameter"() -> (w1115:T2[])
            n513 = local read "colors"() -> (w1113:u32[])
            n514 = for {
              shift-right: [w1124] -> w1114
              shift-left: w1112 -> [w1125]
              tunnel: w1115 -> [w1123] mode=indexing
              tunnel: w1113 -> [w1122] mode=indexing
              n515 = Insert Into Map(map in=w1125, key=w1123, value=w1122) -> (map out=w1124:map{T2, u32})  [unwired: 2 out]
            }
            n516 = local write "color Map"(w1114) -> ()
            n517 = Look In Map(map=w1114, key=3-lorentzian-parameters."ζ" ("Plost: sweep window")) -> (value=w1116:u32)  [unwired: 1 in, 1 out]
            n518 = Look In Map(map=w1114, key=3-lorentzian-parameters."τ1" ("Plost: sweep window")) -> (value=w1117:u32)  [unwired: 1 in, 1 out]
            n519 = Look In Map(map=w1114, key=3-lorentzian-parameters."τS" ("Plost: sweep window")) -> (value=w1118:u32)  [unwired: 1 in, 1 out]
            n520 = Look In Map(map=w1114, key=3-lorentzian-parameters."τN" ("Plost: sweep window")) -> (value=w1119:u32)  [unwired: 1 in, 1 out]
            n521 = Look In Map(map=w1114, key=3-lorentzian-parameters."τC" ("Plost: sweep window")) -> (value=w1120:u32)  [unwired: 1 in, 1 out]
            n522 = Look In Map(map=w1114, key=3-lorentzian-parameters."κ0" ("Plost: sweep window")) -> (value=w1121:u32)  [unwired: 1 in, 1 out]
            n523 = property on="ζ" class="Slide (strict)"("Fill Color"=w1116) -> ()  [unwired: 2 in, 2 out]
            n524 = property on="T1" class="Slide (strict)"("Fill Color"=w1117) -> ()  [unwired: 2 in, 2 out]
            n525 = property on="τS" class="Slide (strict)"("Fill Color"=w1118) -> ()  [unwired: 2 in, 2 out]
            n526 = property on="τN" class="Slide (strict)"("Fill Color"=w1119) -> ()  [unwired: 2 in, 2 out]
            n527 = property on="τC" class="Slide (strict)"("Fill Color"=w1120) -> ()  [unwired: 2 in, 2 out]
            n528 = property on="κ0" class="Slide (strict)"("Fill Color"=w1121) -> ()  [unwired: 2 in, 2 out]
          }
          frame "interface: update plot colors cursors" {
            w1131 = T2[] [enum."m1", enum."m2", enum."m3"] items=["ζ", "τ1", "τS", "τN", "τC", "κ0", "m1", "m2", "m3", "T (K)", "B (T)", "θ (deg)", "side (S|R)", "set of (B|T)", "Re(offset)", "Im(offset)", "στ1", "στ1-", "στ1+", "στS", "στS-", "στS+", "στN", "στN-", "στN+", "τ11", "τ12", "τ21", "τ22", "τN1", "τN2"]
            w1129 = T2[] [enum."T (K)", enum."B (T)", enum."θ (deg)"] items=["ζ", "τ1", "τS", "τN", "τC", "κ0", "m1", "m2", "m3", "T (K)", "B (T)", "θ (deg)", "side (S|R)", "set of (B|T)", "Re(offset)", "Im(offset)", "στ1", "στ1-", "στ1+", "στS", "στS-", "στS+", "στN", "στN-", "στN+", "τ11", "τ12", "τ21", "τ22", "τN1", "τN2"]
            n529 = local read "parameter map"() -> (w1144:map{T2, dbl})
            n530 = local read "cursor x selector"() -> (w1132:map{T2, dbl})
            n531 = local read "X selector"() -> (w1133:T2)
            n532 = local read "T (K)"() -> (w1134:dbl)
            n533 = local read "θ (deg)"() -> (w1139:dbl)
            n534 = local read "B (T)"() -> (w1138:dbl)
            n535 = local read "T (K)"() -> (w1137:dbl)
            n536 = call "3-lorentzian-heat-response -- V4.vi"("action"=3-lorentzian-heat-response_action."calc m1m2m3", "Map IN"=w1144) -> ("Map OUT"=w1140:map{T2, dbl})  [unwired: 7 in, 2 out]
            n537 = local read "parameter"() -> (w1145:T2[])
            n538 = local read "cursor index map"() -> (w1136:map{T2, i32})
            n539 = Look In Map(map=w1132, key=w1133, default value=w1134) -> (value=w1135:dbl)  [unwired: 1 out]
            n540 = Build Array(w1137, w1138, w1139) -> (w1127:dbl[])
            n541 = Build Array (concatenate)(w1145, w1131) -> (w1143:T2[])
            n542 = for {
              shift-right: [w1148] -> w1141
              shift-left: w1140 -> [w1149]
              tunnel: w1129 -> [w1147] mode=indexing
              tunnel: w1127 -> [w1146] mode=indexing
              n543 = Insert Into Map(map in=w1149, key=w1147, value=w1146) -> (map out=w1148:map{T2, dbl})  [unwired: 2 out]
            }
            n544 = for {
              tunnel: w1135 -> [w1157]
              tunnel: w1126 -> [w1156]
              tunnel: w1143 -> [w1152] mode=indexing
              tunnel: w1136 -> [w1154]
              shift-right: [w1151] -> _
              shift-left: w1140 -> [w1151]
              n545 = Look In Map(map=w1151, key=w1152) -> (value=w1150:dbl)  [unwired: 1 in, 1 out]
              n546 = Look In Map(map=w1154, key=w1152) -> (value=w1153:i32)  [unwired: 1 in, 1 out]
              n547 = call "replace cursor - plot ref - V2.vi"("Plot ref in"=w1156, "new X"=w1157, "new  Y"=w1150, "cursor index"=w1153, "cursor action"=cursor_action."write") -> ()  [unwired: 11 in, 4 out]
            }
            n548 = call "string parse mathematica assosiated array.vi"("action"=mathematica_string_map_action."create string" ("derivative"), "map IN"=w1141) -> ("String OUT"=w1142:string)  [unwired: 8 in, 1 out]
            n549 = local write "String"(w1142) -> ()
          }
          frame "interface: plot colors update m1m2m3 cursors" {
            w1159 = T2[] [enum."m1", enum."m2", enum."m3"] items=["ζ", "τ1", "τS", "τN", "τC", "κ0", "m1", "m2", "m3", "T (K)", "B (T)", "θ (deg)", "side (S|R)", "set of (B|T)", "Re(offset)", "Im(offset)", "στ1", "στ1-", "στ1+", "στS", "στS-", "στS+", "στN", "στN-", "στN+", "τ11", "τ12", "τ21", "τ22", "τN1", "τN2"]
            n550 = local read "parameter map"() -> (w1167:map{T2, dbl})
